vi "Obtain Log Queue.vi"(8 "error in":errorcluster) -> (0 "error out":errorcluster, 3 "queue out":refnum<queue>)   [LabVIEW 2016, in "Huskie Swerve.lvlib"]
uses:
  Refname/Huskie Board.ctl
  Refname/Refname to String (Huskie Board).vi
  Huskie Swerve.lvlib
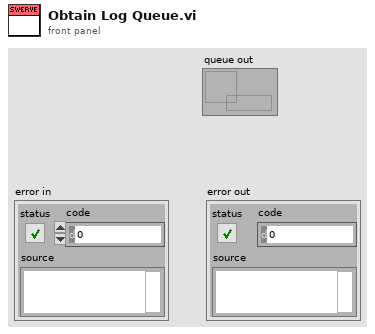
[diagram p1: front panel]
types:
  T1 = typedef "Huskie Swerve.lvlib/Huskie Board.ctl" = enum16{"Huskie Board", "Log Queue", ""}
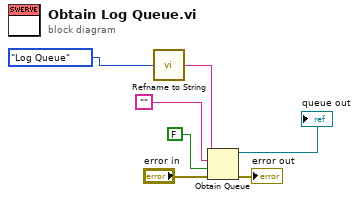
[diagram p0: block diagram]
diagram:
  n1 = call-poly "Refname to String.vi"("Enum"=Huskie_Board."Log Queue") -> ("resulting string"=w2:string)
  n2 = Obtain Queue(name (unnamed)=w2, element data type="", create if not found? (T)=FALSE, error in (no error)="error in") -> (queue out=→"queue out":refnum<queue>, error out=→"error out":errorcluster)  [unwired: 1 in, 1 out]
